vi "Google form using labview.vi"() -> ()   [LabVIEW 2025]
uses:
  <vilib>/Utility/file.llb/Write Delimited Spreadsheet (string).vi
panel:
  in  "Tab Control":enum32{"BASIC DETAILS"}(tab)
  in  "Name":string="Name"
  in  "ID":string="ID"
  in  "Contact":string="Email"
  in  "OK Button":bool
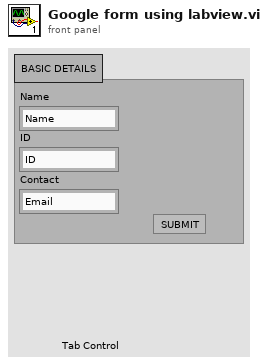
[diagram p1: front panel]
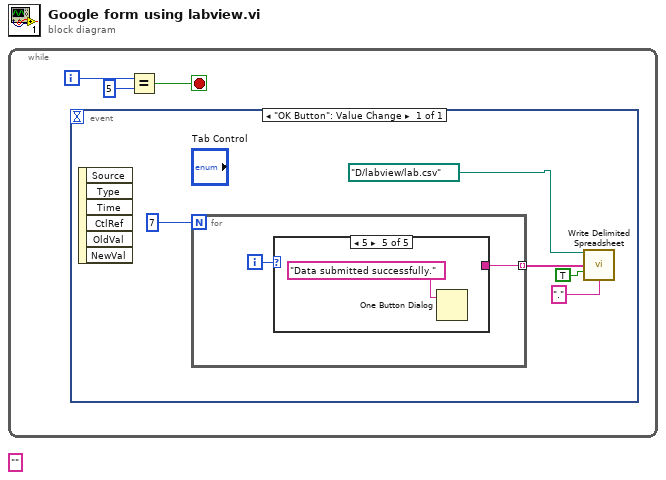
[diagram p0: block diagram]
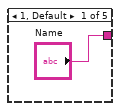
[diagram p2: hidden frame]
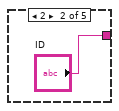
[diagram p3: hidden frame]
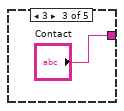
[diagram p4: hidden frame]
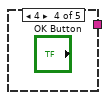
[diagram p5: hidden frame]
diagram:
  (unwired) ""
  n1 = while {
    i -> [w2]
    stop <- w3 stop-if-true
    n2 = event shown="[0] \"OK Button\": Value Change" {
      selector: _ -> [_]
      dyn-events: _ -> [_]
      timeout: _ -> [_]
      event "OK Button": Value Change {
        n3 = event-data() -> ()  [unwired: 1 in, 6 out]
        n4 = for {
          N: 7 -> [_]
          tunnel: [w9] -> w7 mode=indexing
          i -> [w10]
          n5 = case shown="5" w10 {
            tunnel: ["Name" "ID" "Contact" _ _] -> w9
            frame 1, Default {
            }
            frame 2 {
            }
            frame 3 {
            }
            frame 4 {
            }
            frame 5 {
              n6 = One Button Dialog(message="Data submitted successfully.") -> ()  [unwired: 1 in, 1 out]
            }
          }
        }
        n7 = call-poly <vilib>:"Write Delimited Spreadsheet.vi"("file path (dialog if empty)"=path "D:/labview/lab.csv", "1D data"=w7, "append to file? (new file:F)"=TRUE, "delimiter (\\t)"="." ("delimiter (\\t)")) -> ()  [unwired: 10 in, 2 out]
      }
    }
    n8 = Equal?(x=w2, y=5) -> (x = y?=w3:bool)
  }
